vi "Public Wait for Lifecycle State.vi"(8 "error in (no error)":errorcluster, 9 "timeout in ms (-1)":i32=-1, 10 "Lifecycle State":T1, 11 "Mock Process in":refnum<class "Mock Process.lvclass">) -> (0 "error out":errorcluster, 1 "timed out?":bool, 3 "Mock Process out":refnum<class "Mock Process.lvclass">)   [LabVIEW 2020, in "Mock Process.lvclass"]
uses:
  Mock Process.lvclass
  Framework/Process/Process.lvclass
  C:/Users/anton/Documents/GitHub/Triarc-Framework/source/Framework/Process/Process.lvclass
  Framework/Process/Public/Lifecycle/Lifecycle State.ctl
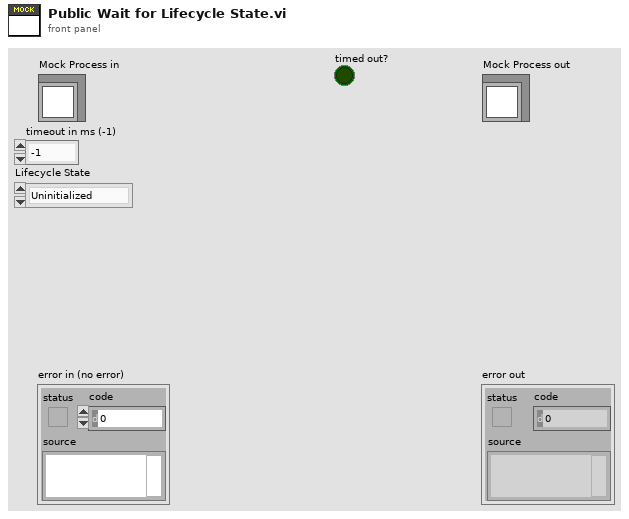
[diagram p1: front panel]
types:
  T1 = typedef "Process.lvclass/Lifecycle State.ctl" = enum16{"Uninitialized", "Initialized", "Started", "Running", "Stopped", "Finished"}
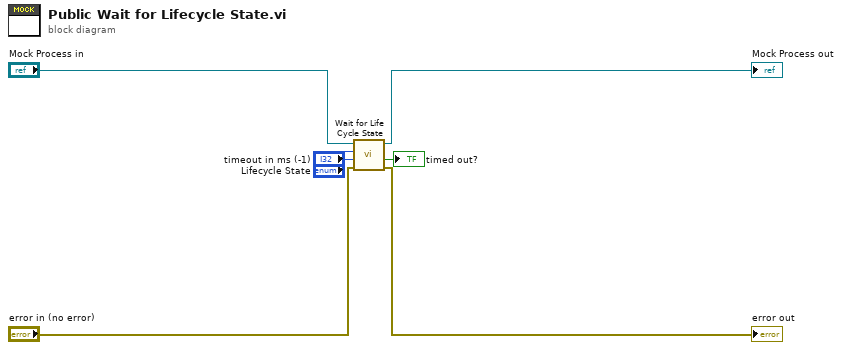
[diagram p0: block diagram]
diagram:
  n1 = call "Wait for Life Cycle State.vi"("error in (no error)"="error in (no error)", "timeout in ms (-1)"="timeout in ms (-1)", "Lifecycle State"="Lifecycle State", "Process In"="Mock Process in") -> ("error out"=→"error out":errorcluster, "timed out?"=→"timed out?":bool, "Process Out"=→"Mock Process out":refnum<class "Mock Process.lvclass">)  [unwired: 5 in]
